vi "Init.vi"(8 "error in (no error)":errorcluster, 11 "uService Template in":refnum<class "TCP Listener.lvclass">) -> (0 "error out":errorcluster, 3 "uService Template out":refnum<class "TCP Listener.lvclass">)   [LabVIEW 2026, in "TALOS.lvlib" / "TCP Listener.lvlib" / "TCP Listener.lvclass"]
uses:
  TCP Listener.lvclass
  C:/LabVIEW Code/TALOS/talos/Ancestor/Ancestor/Ancestor.lvclass
  C:/LabVIEW Code/TALOS/talos/Father of all uServices/Father of all uServices/Father of all uServices.lvclass
  Ancestor/Ancestor/Ancestor.lvclass/Ancestor.ctl
  Father of all uServices/Father of all uServices/Father of all uServices.lvclass/Father of all uServices.ctl
  TCP Listener.lvclass/TCP Listener.ctl
  Support VIs/Substitute Error.vi
  Support VIs/Generate Error.vi
  FGV/Error Memory/Get Error Description.vi
  Support VIs/Get PC name.vi
  Support VIs/Get Class Name.vi
  <vilib>/Utility/error.llb/Clear Errors.vi
  FGV/Error Memory/Error Memory Core.vi
  <vilib>/AdvancedString/Delimited String to 1D String Array.vi
  <vilib>/AdvancedString/Delimited String to 1D String Array (string).vi
  Support VIs/Circus Root Path.vi
  FGV/Error Memory/Error Crt Lvl checker.vi
  FGV/Error Memory/Error Memory Core.vi/40c8088d-b597-4017-91af-faa98e00292e.vi
  FGV/Error Memory/Error Memory Core.vi/d4a3ab98-063c-4e44-b43d-fbdcfe6c2be2.vi
  Support VIs/Global Memory.vi
  <vilib>/Utility/LVClass/Get LV Class Name.vi
  Support VIs/Is in Packed Library.vi
  Support VIs/TALOS Root path.vi
  Support VIs/Read CSV worksheet.vi
  Support VIs/Global Constants.vi
  <vilib>/Utility/error.llb/General Error Handler.vi
  Support VIs/Error Log.vi
  Father of all uServices/Father of all uServices/Father of all uServices.lvclass
  Ancestor/Ancestor/Ancestor.lvclass
  <vilib>/Comparison/Equal/Equal Functor/Equal Functor.lvclass
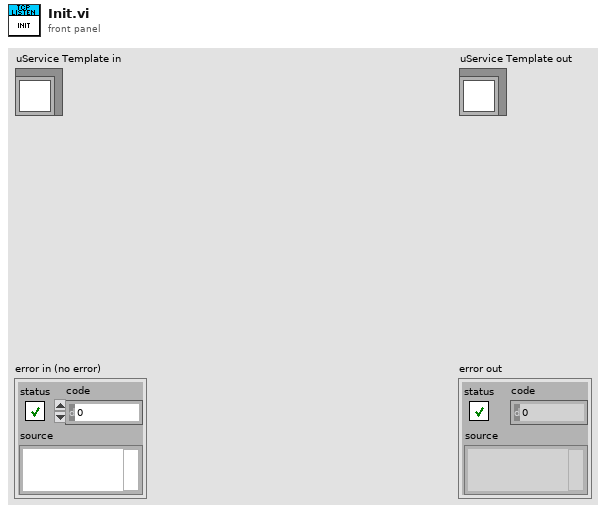
[diagram p1: front panel]
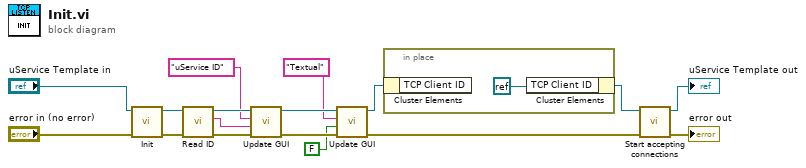
[diagram p0: block diagram]
diagram:
  n1 = call-parent "Init.vi"("error in (no error)"="error in (no error)", "uService Template in"="uService Template in") -> ("error out"=w14:errorcluster, "uService Template out"=w15:refnum<class "TCP Listener.lvclass">)  [unwired: 8 in]
  n2 = call "Read ID.vi"("error in (no error)"=w14, "Ancestor in"=w15) -> ("error out"=w13:errorcluster, "ID"=w10:string, "Ancestor out"=w12:refnum<class "TCP Listener.lvclass">)  [unwired: 7 in]
  n3 = call "Update GUI.vi"("error in (no error)"=w13, "Data"=w10, "GUI Item Name"="uService ID", "uService Template in"=w12) -> ("error out"=w9:errorcluster, "uService Template out"=w7:refnum<class "TCP Listener.lvclass">)  [unwired: 6 in]
  n4 = call "Update GUI.vi"("error in (no error)"=w9, "Data"=FALSE ("Textual"), "GUI Item Name"="Textual", "uService Template in"=w7) -> ("error out"=w4:errorcluster, "uService Template out"=w8:refnum<class "TCP Listener.lvclass">)  [unwired: 6 in]
  n5 = in-place {
    n6 = in-place-cluster #1(w8) -> ()  [unwired: 1 out]
    n7 = in-place-cluster #1("TCP Client ID"=refnum<k0> refnum) -> (w2:refnum<class "TCP Listener.lvclass">)
  }
  n8 = call-dynamic "Start accepting connections.vi"("error in (no error)"=w4, "TCP Listener in"=w2) -> ("error out"=→"error out":errorcluster, "TCP Listener out"=→"uService Template out":refnum<class "TCP Listener.lvclass">)  [unwired: 8 in]
